vi "Test.vi"() -> ()   [LabVIEW 2020]
doc: "This VI is called when test mode begins, and will automatically be terminated when it ends. You can add manual or automatic tests and invoke them from the dashboard."
uses:
  <vilib>/Rock Robotics/WPI/ThirdParty/REV Robotics/REVLib/Typedef/Spark MAX Control Type.ctl
  <vilib>/Rock Robotics/WPI/Utilities/WPI_GetSetVariantRefNum.vi
  981LabViewComponents/2022 Robot Global Data.vi
panel:
  out "test telop\noutput\ncommand":dbl
  out "Error\n(armSetpoint -\n armPosition)":dbl
  out "Commanded\nSet Output":dbl
  out "Premove\nSensor Position":dbl
  out "Sensor Position 2":dbl
  out "armSetpoint":dbl
  out "Sensor Position":dbl
  out "x*y":dbl
  out "element":dbl
  out "x-y":dbl
  out "coerced(x) 2":dbl
  out "Position Error 2":dbl
  out "Position Error":dbl
  in  "PID Zero Constants":T1
  out "Status Plot":dbl[](graph)
  out "YRPHfH":T2
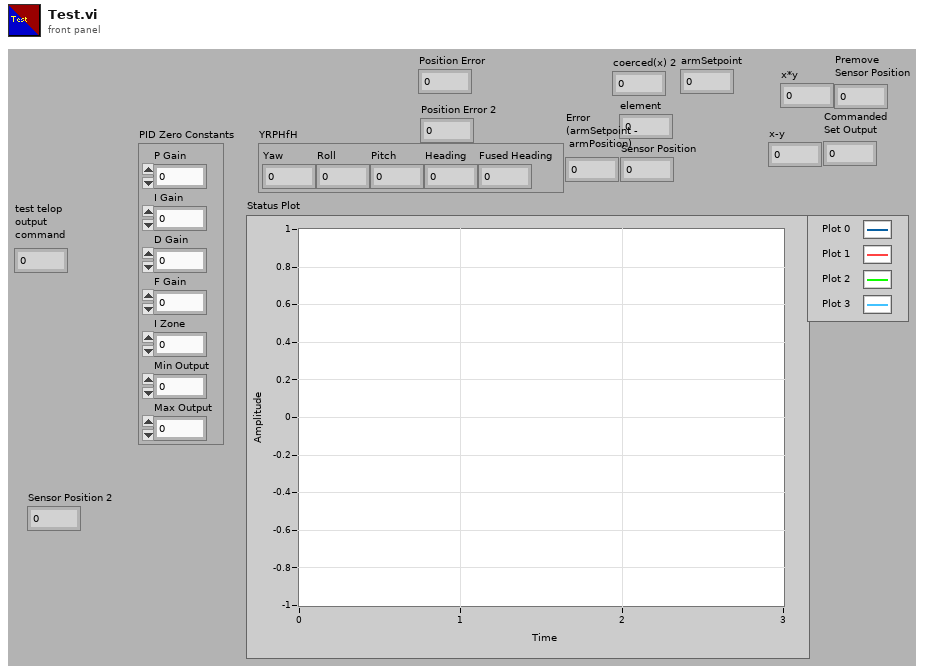
[diagram p1: front panel]
types:
  T1 = cluster{"P Gain":dbl, "I Gain":dbl, "D Gain":dbl, "F Gain":dbl, "I Zone":dbl, "Min Output":dbl, "Max Output":dbl}
  T2 = cluster{"Yaw":dbl, "Roll":dbl, "Pitch":dbl, "Heading":dbl, "Fused Heading":dbl}
  T3 = typedef "WPI_JoystickDevRef.ctl" = cluster{"Device":T4}
  T4 = typedef "WPI_JoystickDeviceEnum.ctl" = enum16{"USB 0", "USB 1", "USB 2", "USB 3", "USB 4", "USB 5"}
  T5 = typedef "WPI_MotorControlDeviceRef.ctl" = cluster{"DeviceStatus":errorcluster, "Type":T6, "PWM":cluster{"PWM Channel":T7, "DeadBand":T8}, "CAN":cluster{"Device Number":u8, "SetOutput VI Ref":variant, "GetOutput VI Ref":variant, "Enable VI Ref":variant, "Disable VI Ref":variant, "Data":variant}, "Invert":bool, "DIO PWM":cluster{"PWM \"Enable\" Channel":T7, "DIOChannel":T9, "PWM Rate":dbl}}
  T6 = typedef "WPI_MotorControlType.ctl" = enum16{"PWM", "CAN", "DIO PWM"}
  T7 = typedef "FPGA_DIOPWMChannel.ctl" = enum8{"PWM 0", "PWM 1", "PWM 2", "PWM 3", "PWM 4", "PWM 5", "PWM 6", "PWM 7", "PWM 8", "PWM 9", "PWM MXP 0", "PWM MXP 1", "PWM MXP 2", "PWM MXP 3", "PWM MXP 4", "PWM MXP 5", "PWM MXP 6", "PWM MXP 7", "PWM MXP 8", "PWM MXP 9", "Invalid"}
  T8 = typedef "WPI_PWMDeadband.ctl" = cluster{"Name":string, "maxPositivePwm":i32, "minPositivePwm":i32, "centerPwm":i32, "maxNegativePwm":i32, "minNegativePwm":i32, "angularRange":u16}
  T9 = typedef "FPGA_DIOChannel.ctl" = enum8{"DIO 0", "DIO 1", "DIO 2", "DIO 3", "DIO 4", "DIO 5", "DIO 6", "DIO 7", "DIO 8", "DIO 9", "DIO MXP 0", "DIO MXP 1", "DIO MXP 2", "DIO MXP 3", "DIO MXP 4", "DIO MXP 5", "DIO MXP 6", "DIO MXP 7", "DIO MXP 8", "DIO MXP 9", "DIO MXP 10", "DIO MXP 11", "DIO MXP 12", "DIO MXP 13", "DIO MXP 14", "DIO MXP 15", "SPI Port CS1", "SPI Port CS2", "SPI Port CS3", "SPI Port MISO", "SPI Port MOSI", "Invalid"}
  T10 = typedef "Spark MAX Control Type.ctl" = enum16{"Percent VBus", "Voltage", "Velocity", "Position", "Smart Motion", "Current", "Smart Velocity"}
  T11 = cluster{"P Gain":bool, "I Gain":bool, "D Gain":bool, "F Gain":bool, "I Zone":bool, "Min Output":bool, "Max Output":bool}
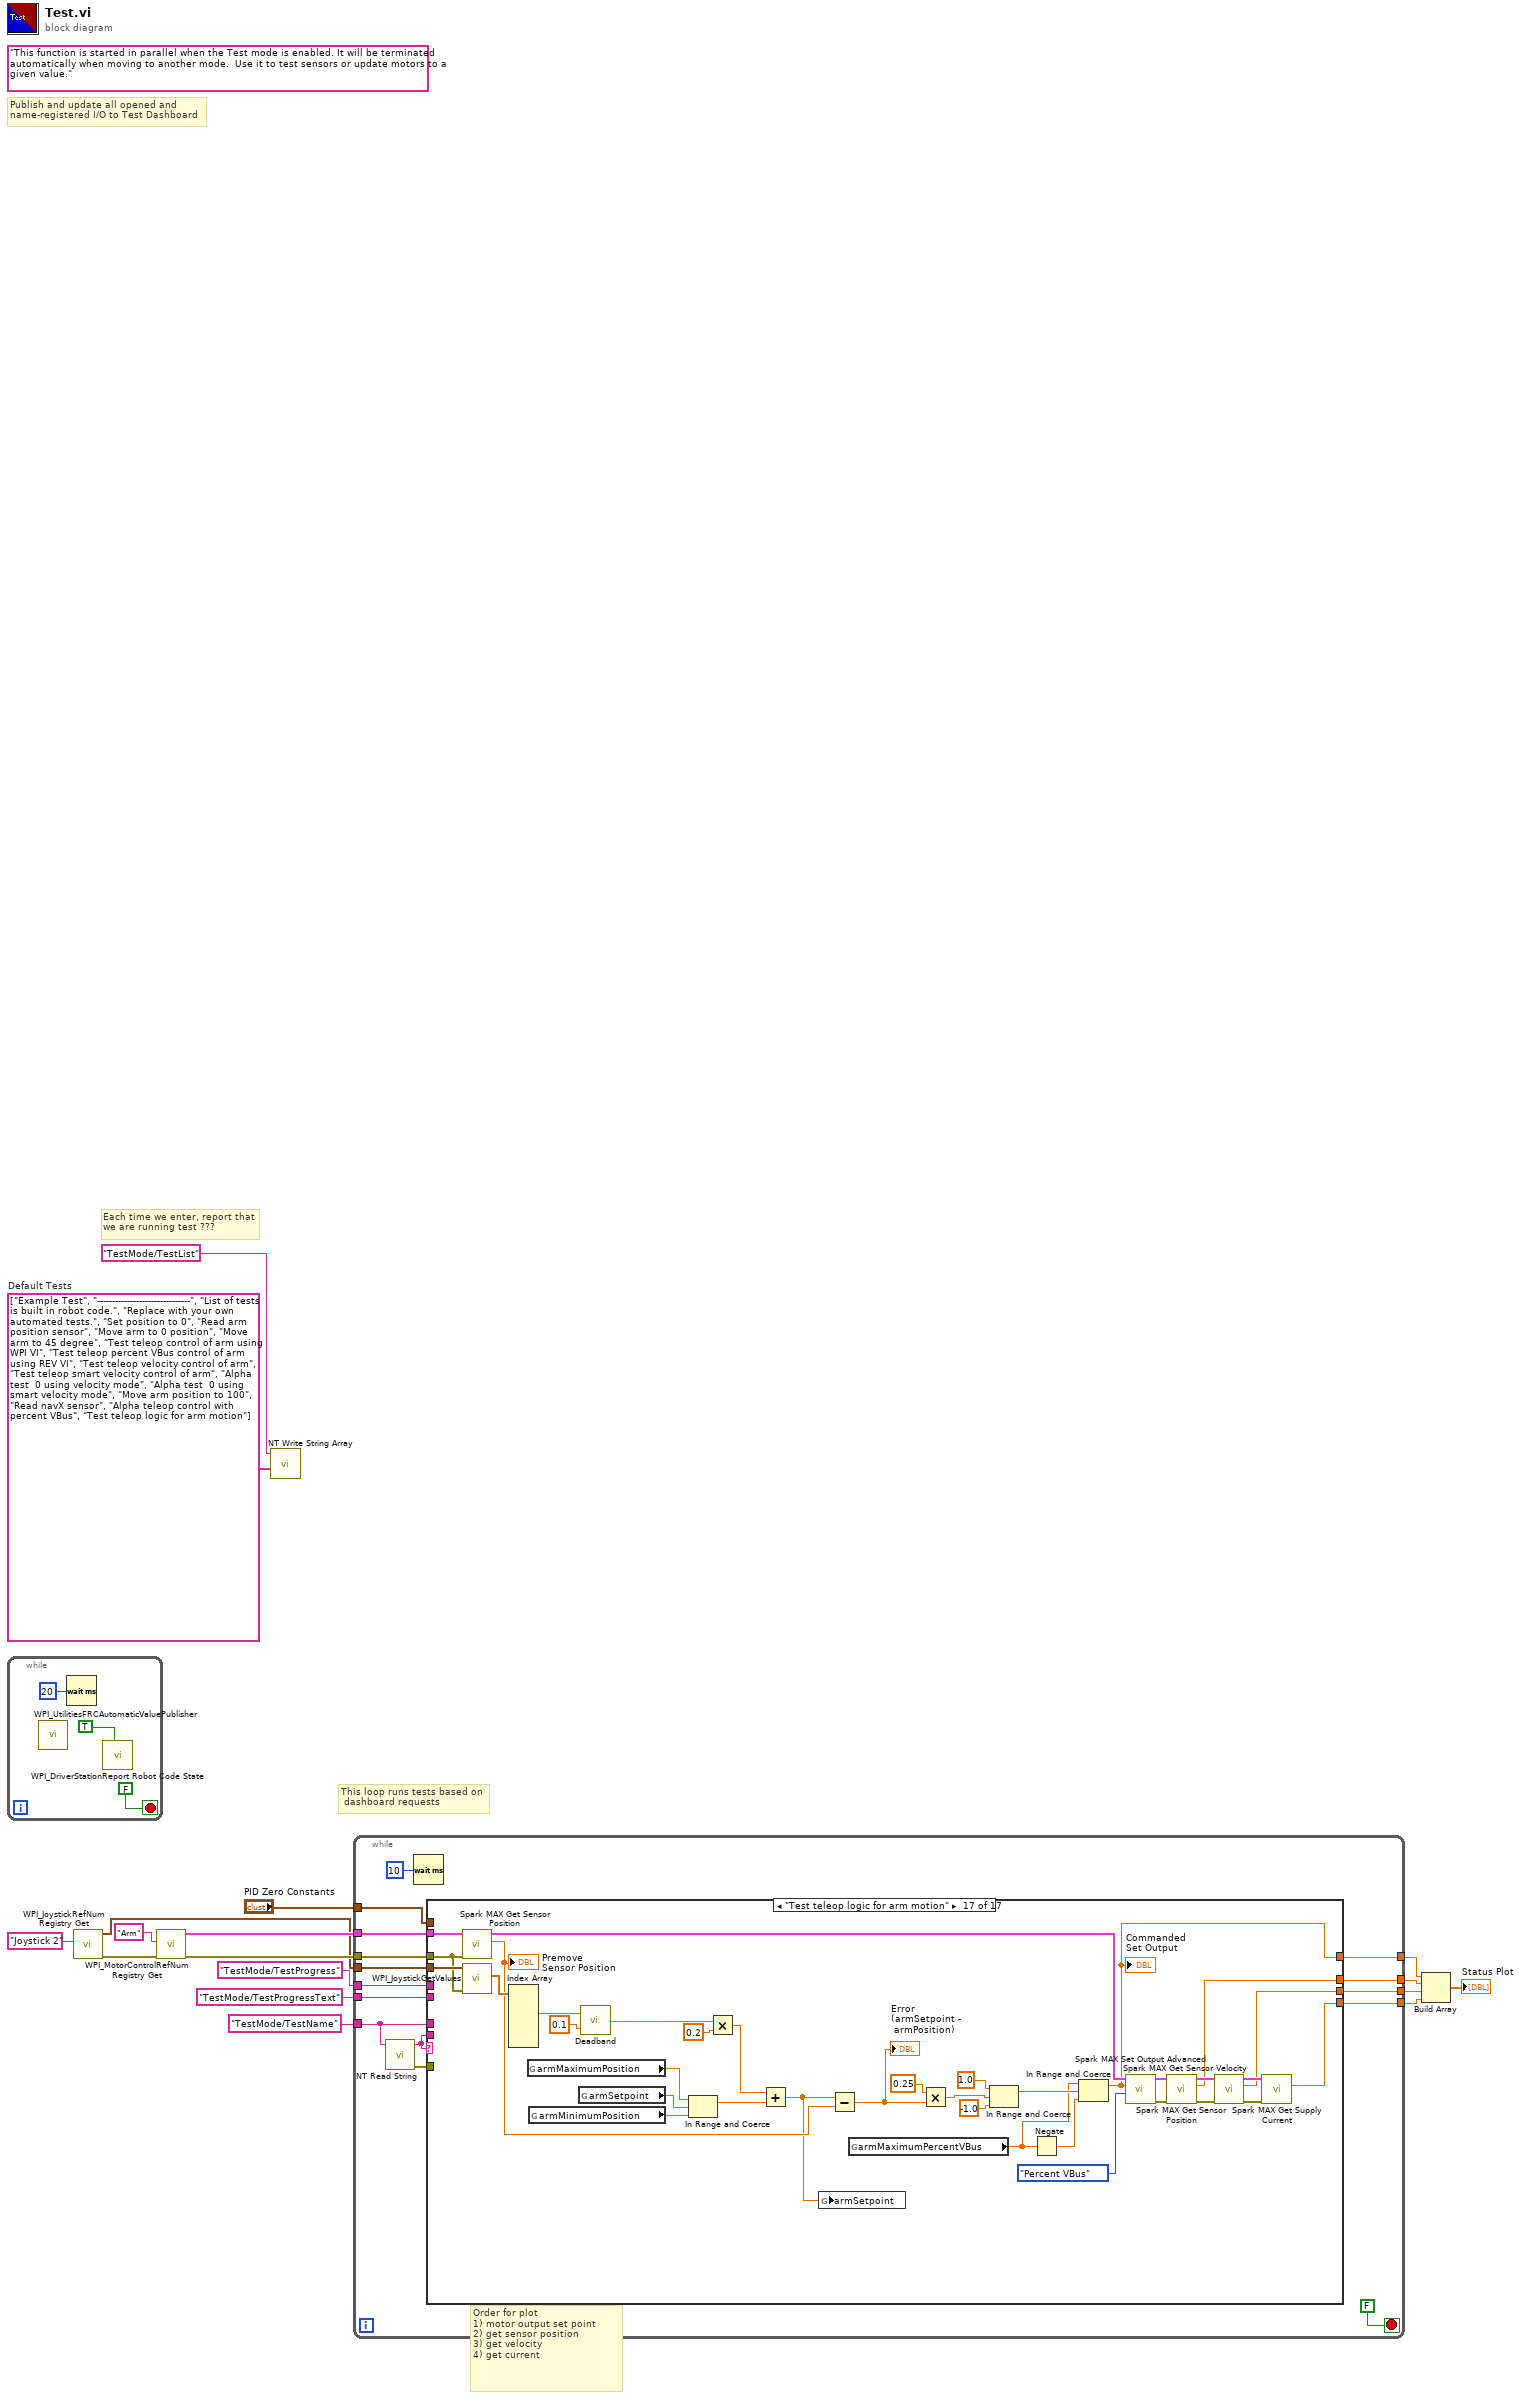
[diagram p0: block diagram]
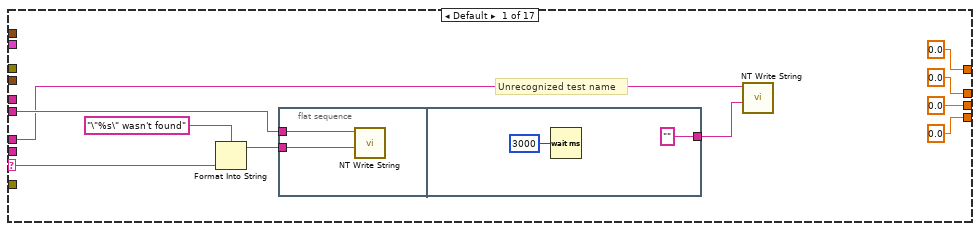
[diagram p2: hidden frame]
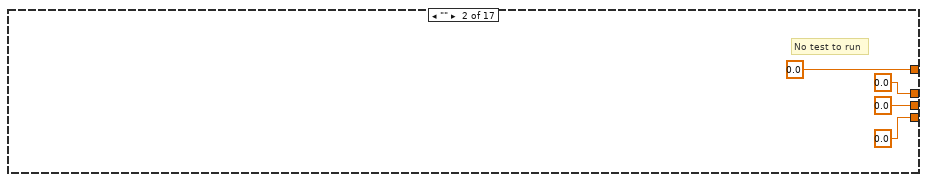
[diagram p3: hidden frame]
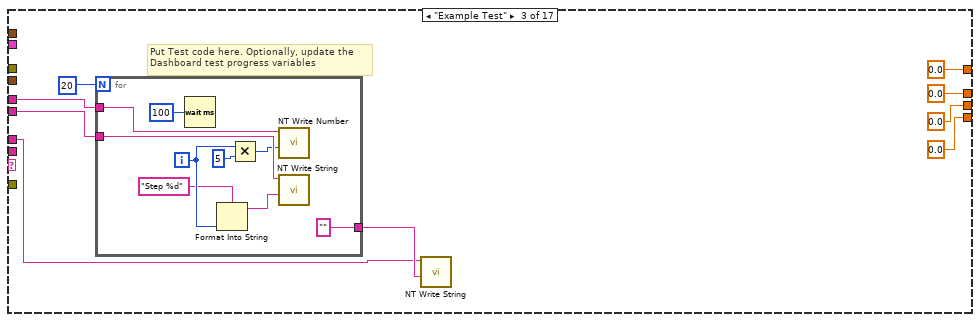
[diagram p4: hidden frame]
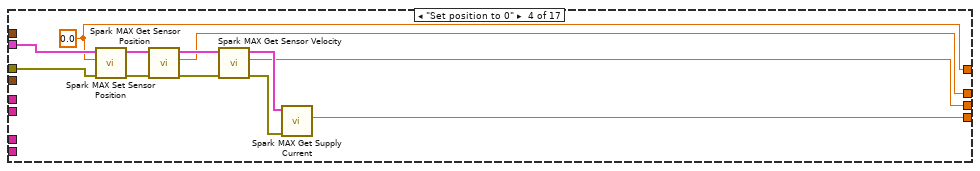
[diagram p5: hidden frame]
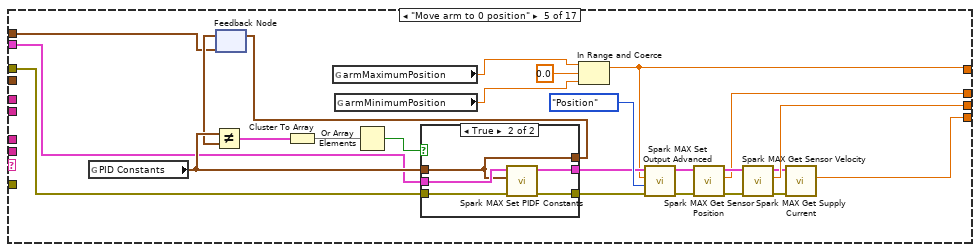
[diagram p6: hidden frame]
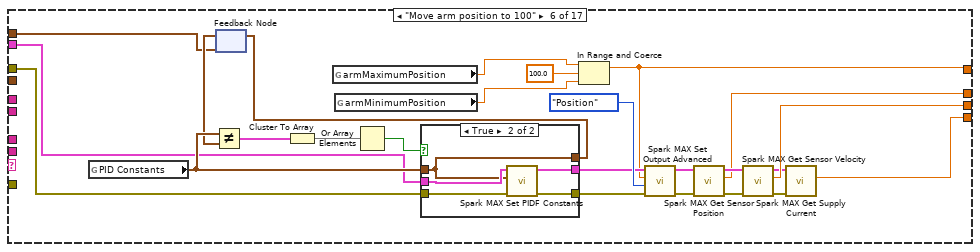
[diagram p8: hidden frame]
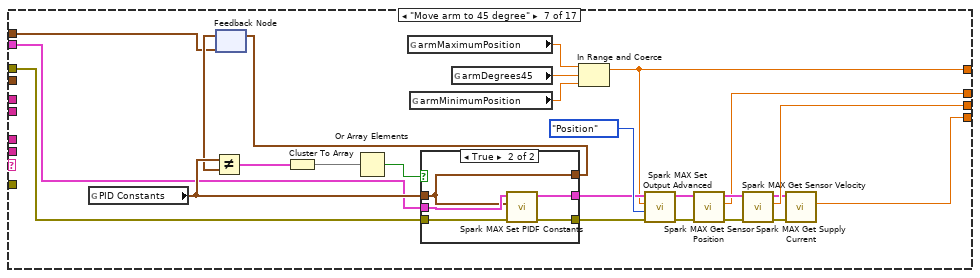
[diagram p10: hidden frame]
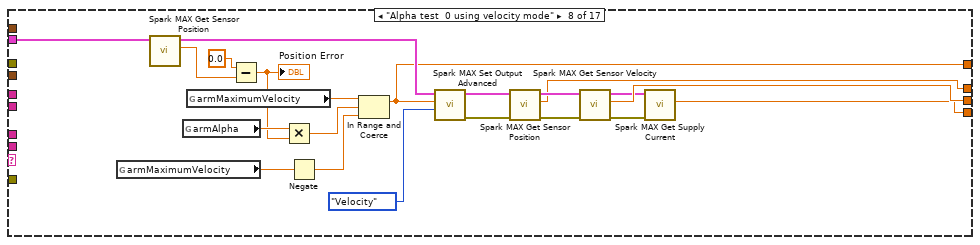
[diagram p12: hidden frame]
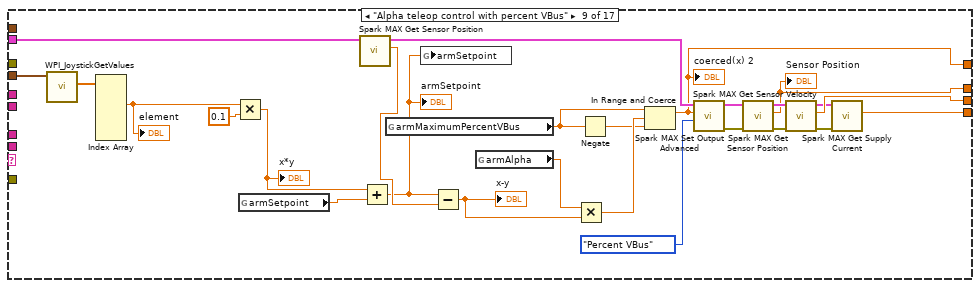
[diagram p13: hidden frame]
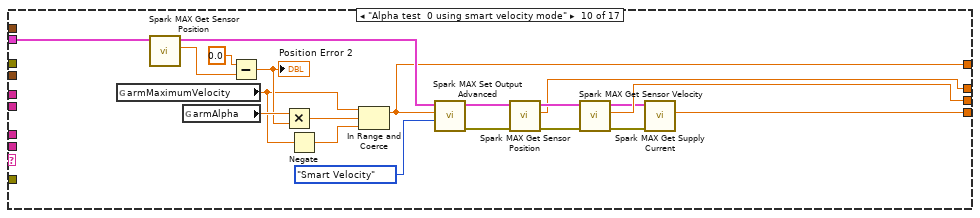
[diagram p14: hidden frame]
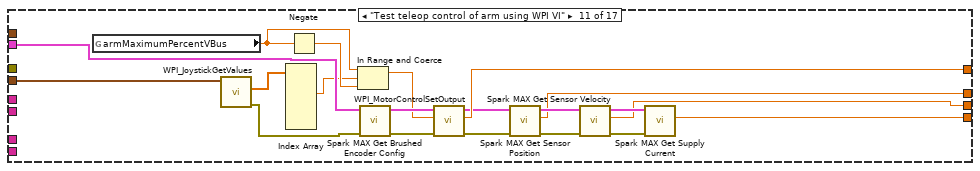
[diagram p15: hidden frame]
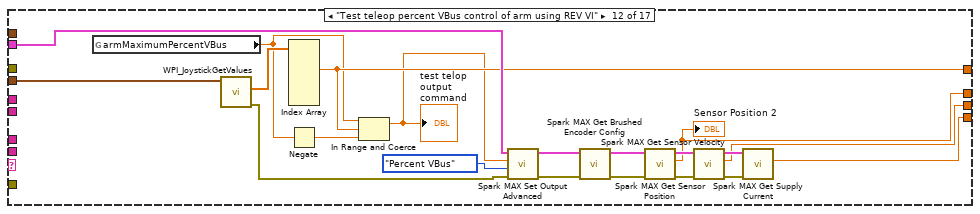
[diagram p16: hidden frame]
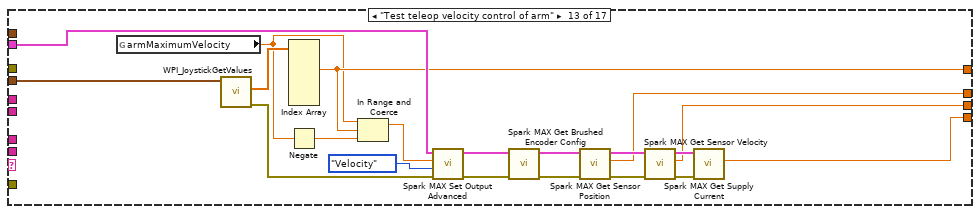
[diagram p17: hidden frame]
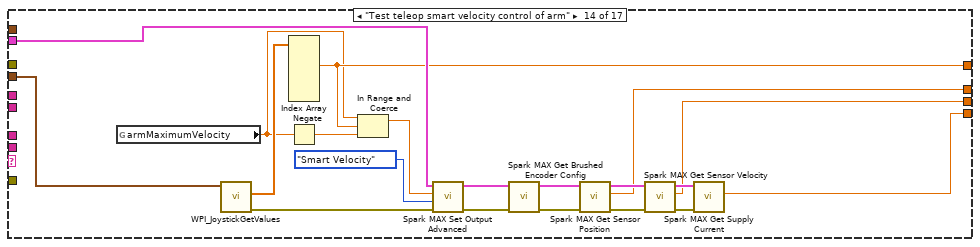
[diagram p18: hidden frame]
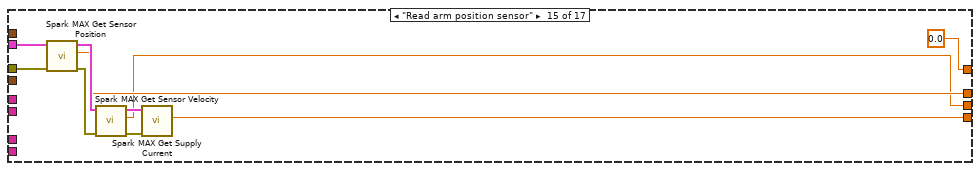
[diagram p19: hidden frame]
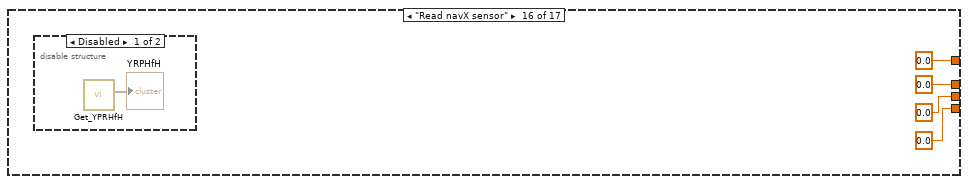
[diagram p20: hidden frame]
diagram:
  w14 = string[] ["Example Test", "-------------------------------", "List of tests is built in robot code.", "Replace with your own automated tests.", "Set position to 0", "Read arm position sensor", "Move arm to 0 position", "Move arm to 45 degree", "Test teleop control of arm using WPI VI", "Test teleop percent VBus control of arm using REV VI", "Test teleop velocity control of arm", "Test teleop smart velocity control of arm", "Alpha test  0 using velocity mode", "Alpha test  0 using smart velocity mode", "Move arm position to 100", "Read navX sensor", "Alpha teleop control with percent VBus", "Test teleop logic for arm motion"]  # Default Tests
  (unwired) "This function is started in parallel when the Test mode is enabled. It will be terminated automatically when moving to another mode.  Use it to test sensors or update motors to a given value."
  # "This loop runs tests based on \n dashboard requests"
  # "Publish and update all opened and\nname-registered I/O to Test Dashboard"
  # "Each time we enter, report that\nwe are running test ???"
  n1 = while {
    stop <- FALSE stop-if-true
    n2 = call <vilib>:"WPI_UtilitiesFRCAutomaticValuePublisher.vi"() -> ()  [unwired: 12 in]
    n3 = Wait (ms)(milliseconds to wait=u32 20) -> ()  [unwired: 1 out]
    n4 = call <vilib>:"WPI_DriverStationReport Robot Code State.vi"("Test"=TRUE ("Autonomous")) -> ()  [unwired: 10 in, 1 out]
  }
  n5 = call <vilib>:"WPI_JoystickRefNum Registry Get.vi"("refnum name"="Joystick 2") -> ("error out"=w1:errorcluster, "JoystickDevRef"=w7:T3)  [unwired: 1 in, 8 out]
  n6 = call <vilib>:"WPI_MotorControlRefNum Registry Get.vi"("error in (no error)"=w1, "refnum name"="Arm") -> ("error out"=w9:errorcluster, "MotorControlDevRef"=w10:T5)  [unwired: 8 in]
  n7 = call <vilib>:"NT Write String Array.vi"("String Array"=w14, "Name"="TestMode/TestList") -> ()  [unwired: 9 in, 1 out]
  n8 = while {
    tunnel: "TestMode/TestName" ("Name") -> [w30]
    tunnel: "TestMode/TestProgressText" ("Name") -> [w33]
    tunnel: "TestMode/TestProgress" ("Name") -> [w32]
    tunnel: w7 -> [w28]
    tunnel: w10 -> [w27]
    tunnel: w9 -> [w26]
    tunnel: "PID Zero Constants" -> [w25]
    tunnel: [w24] -> w5
    tunnel: [w23] -> w2
    tunnel: [w22] -> w4
    tunnel: [w21] -> w3
    stop <- FALSE stop-if-true
    # "Order for plot\n1) motor output set point\n2) get sensor position\n3) get velocity\n4) get current"
    n9 = call <vilib>:"NT Read String.vi"("Name"=w30) -> ("error out"=w29:errorcluster, "String"=w31:string)  [unwired: 9 in]
    n10 = Wait (ms)(milliseconds to wait=u32 10) -> ()  [unwired: 1 out]
    n11 = case shown="\"Test teleop logic for arm motion\"" w31 {
      selector: w31 -> [w44 _ _ _ _ _ _ _ _ _ _ _ _ _ _ _ _]
      tunnel: w30 -> [w41 _ w58 _ _ _ _ _ _ _ _ _ _ _ _ _ _]
      tunnel: w33 -> [w45 _ w61 _ _ _ _ _ _ _ _ _ _ _ _ _ _]
      tunnel: w32 -> [_ _ w62 _ _ _ _ _ _ _ _ _ _ _ _ _ _]
      tunnel: w31 -> [_ _ _ _ _ _ _ _ _ _ _ _ _ _ _ _ _]
      tunnel: w29 -> [_ _ _ _ _ _ _ _ _ _ _ _ _ _ _ _ _]
      tunnel: [0.0 ("armMaximumPosition") 0.0 ("armMaximumPosition") 0.0 ("armMaximumPosition") w81 w93 w126 w159 w183 w213 w231 w268 w273 w291 w312 0.0 ("armMaximumPosition") 0.0 ("armMaximumPosition") w349] -> w24
      tunnel: [0.0 ("Sensor Position") 0.0 ("Sensor Position") 0.0 ("Sensor Position") w73 w92 w125 w158 w200 w226 w246 w256 w270 w295 w315 w332 0.0 ("Sensor Position") w348] -> w23
      tunnel: [0.0 ("Sensor Velocity") 0.0 ("Sensor Velocity") 0.0 ("Sensor Velocity") w72 w91 w124 w157 w199 w225 w245 w255 w275 w294 w314 w331 0.0 ("Sensor Velocity") w347] -> w22
      tunnel: [0.0 ("Sensor Position") 0.0 ("Sensor Position") 0.0 ("Sensor Position") w80 w87 w120 w153 w196 w222 w242 w254 w282 w302 w322 w330 0.0 ("Sensor Position") w346] -> w21
      tunnel: w28 -> [_ _ _ _ _ _ _ _ w207 _ w267 w285 w305 w325 _ _ w374]
      tunnel: w27 -> [_ _ _ w83 w86 w119 w152 w191 w217 w237 w266 w284 w304 w324 w338 _ w373]
      tunnel: w26 -> [_ _ _ w82 w85 w118 w151 _ _ _ _ _ _ _ w339 _ w372]
      tunnel: w25 -> [_ _ _ _ w84 w117 w150 _ _ _ _ _ _ _ _ _ _]
      frame Default {
        # "Unrecognized test name"
        n12 = Format Into String(format string="\"%s\" wasn't found" ("Name"), w44) -> (resulting string=w43:string)  [unwired: 2 in, 1 out]
        n13 = flat-sequence {
          tunnel: w45 -> [w46]
          tunnel: w43 -> [w47]
          tunnel: ["" ("Name")] -> w40
          frame #0 {
            n14 = call <vilib>:"NT Write String.vi"("String"=w47, "Name"=w46) -> ()  [unwired: 9 in, 1 out]
          }
          frame #1 {
            n15 = Wait (ms)(milliseconds to wait=u32 3000) -> ()  [unwired: 1 out]
          }
        }
        n16 = call <vilib>:"NT Write String.vi"("String"=w40, "Name"=w41) -> ()  [unwired: 9 in, 1 out]
      }
      frame "" {
        # "No test to run"
      }
      frame "Example Test" {
        # "Put Test code here. Optionally, update the\nDashboard test progress variables"
        n17 = for {
          N: 20 -> [_]
          tunnel: w62 -> [w71]
          tunnel: w61 -> [w69]
          tunnel: ["" ("String")] -> w59
          i -> [w66]
          n18 = Wait (ms)(milliseconds to wait=u32 100) -> ()  [unwired: 1 out]
          n19 = Format Into String(format string="Step %d", w66) -> (resulting string=w64:string)  [unwired: 2 in, 1 out]
          n20 = Multiply(x=w66, y=u32 5 ("milliseconds to wait")) -> (x*y=w67:u32)
          n21 = call <vilib>:"NT Write Number.vi"("Numeric"=w67, "Name"=w71) -> ()  [unwired: 9 in, 1 out]
          n22 = call <vilib>:"NT Write String.vi"("String"=w64, "Name"=w69) -> ()  [unwired: 9 in, 1 out]
        }
        n23 = call <vilib>:"NT Write String.vi"("String"=w59, "Name"=w58) -> ()  [unwired: 9 in, 1 out]
      }
      frame "Set position to 0" {
        w81 = 0.0 ("Position")
        n24 = call <vilib>:"Spark MAX Set Sensor Position.vi"("error in"=w82, "Position"=w81, "MotorControlDeviceRef"=w83) -> ("error out"=w79:errorcluster, "MotorControlDeviceRef"=w78:T5)  [unwired: 7 in]
        n25 = call <vilib>:"Spark MAX Get Sensor Position.vi"("error in (no error)"=w79, "MotorControlDevRef in"=w78) -> ("error out"=w77:errorcluster, "Sensor Position"=w73:dbl, "MotorControlDevRef out"=w76:T5)  [unwired: 6 in, 1 out]
        n26 = call <vilib>:"Spark MAX Get Sensor Velocity.vi"("error in (no error)"=w77, "MotorControlDevRef in"=w76) -> ("error out"=w74:errorcluster, "Sensor Velocity"=w72:dbl, "MotorControlDevRef out"=w75:T5)  [unwired: 6 in, 1 out]
        n27 = call <vilib>:"Spark MAX Get Supply Current.vi"("error in (no error)"=w74, "MotorControlDevRef in"=w75) -> ("Current"=w80:dbl)  [unwired: 6 in, 3 out]
      }
      frame "Move arm to 0 position" {
        n28 = global read "2022 Robot Global Data.vi" "PID Constants"() -> (w99:T1)
        n29 = feedback #1(w84) -> (w98:T1)
        n30 = Not Equal?(x=w99, y=w98) -> (x != y?=w97:T11)
        n31 = Cluster To Array(cluster=w97) -> (array=w96:bool[])
        n32 = global read "2022 Robot Global Data.vi" "armMaximumPosition"() -> (w107:dbl)
        n33 = global read "2022 Robot Global Data.vi" "armMinimumPosition"() -> (w106:dbl)
        n34 = Or Array Elements(Boolean array=w96) -> (logical OR=w95:bool)
        n35 = case shown="True" w95 {
          tunnel: w85 -> [w109 w116]
          tunnel: w86 -> [w110 w115]
          tunnel: [w109 w114] -> w101
          tunnel: [w110 w113] -> w100
          tunnel: w99 -> [w111 w112]
          tunnel: [w111 w112] -> w94
          frame False {
          }
          frame True {
            n36 = call <vilib>:"Spark MAX Set PIDF Constants.vi"("error in"=w116, "PID Constants"=w112, "MotorControlDeviceRef"=w115) -> ("error out"=w114:errorcluster, "MotorControlDeviceRef"=w113:T5)  [unwired: 7 in]
          }
        }
        n37 = feedback-in #1(w94) -> ()
        n38 = In Range and Coerce(upper limit=w107, x=0.0, lower limit=w106) -> (coerced(x)=w93:dbl)  [unwired: 1 out]
        n39 = call <vilib>:"Spark MAX Set Output Advanced.vi"("error in (no error)"=w101, "Control Mode"=Spark_MAX_Control_Type."Position", "Setpoint"=w93, "MotorControlDevRef"=w100) -> ("error out"=w105:errorcluster, "MotorControlDevRef"=w103:T5)  [unwired: 6 in]
        n40 = call <vilib>:"Spark MAX Get Sensor Position.vi"("error in (no error)"=w105, "MotorControlDevRef in"=w103) -> ("error out"=w104:errorcluster, "Sensor Position"=w92:dbl, "MotorControlDevRef out"=w102:T5)  [unwired: 6 in, 1 out]
        n41 = call <vilib>:"Spark MAX Get Sensor Velocity.vi"("error in (no error)"=w104, "MotorControlDevRef in"=w102) -> ("error out"=w88:errorcluster, "Sensor Velocity"=w91:dbl, "MotorControlDevRef out"=w89:T5)  [unwired: 6 in, 1 out]
        n42 = call <vilib>:"Spark MAX Get Supply Current.vi"("error in (no error)"=w88, "MotorControlDevRef in"=w89) -> ("Current"=w87:dbl)  [unwired: 6 in, 3 out]
      }
      frame "Move arm position to 100" {
        n43 = global read "2022 Robot Global Data.vi" "PID Constants"() -> (w132:T1)
        n44 = feedback #2(w117) -> (w131:T1)
        n45 = Not Equal?(x=w132, y=w131) -> (x != y?=w130:T11)
        n46 = Cluster To Array(cluster=w130) -> (array=w129:bool[])
        n47 = global read "2022 Robot Global Data.vi" "armMaximumPosition"() -> (w140:dbl)
        n48 = global read "2022 Robot Global Data.vi" "armMinimumPosition"() -> (w139:dbl)
        n49 = Or Array Elements(Boolean array=w129) -> (logical OR=w128:bool)
        n50 = case shown="True" w128 {
          tunnel: w118 -> [w142 w149]
          tunnel: w119 -> [w143 w148]
          tunnel: [w142 w147] -> w134
          tunnel: [w143 w146] -> w133
          tunnel: w132 -> [w144 w145]
          tunnel: [w144 w145] -> w127
          frame False {
          }
          frame True {
            n51 = call <vilib>:"Spark MAX Set PIDF Constants.vi"("error in"=w149, "PID Constants"=w145, "MotorControlDeviceRef"=w148) -> ("error out"=w147:errorcluster, "MotorControlDeviceRef"=w146:T5)  [unwired: 7 in]
          }
        }
        n52 = feedback-in #2(w127) -> ()
        n53 = In Range and Coerce(upper limit=w140, x=100.0, lower limit=w139) -> (coerced(x)=w126:dbl)  [unwired: 1 out]
        n54 = call <vilib>:"Spark MAX Set Output Advanced.vi"("error in (no error)"=w134, "Control Mode"=Spark_MAX_Control_Type."Position", "Setpoint"=w126, "MotorControlDevRef"=w133) -> ("error out"=w138:errorcluster, "MotorControlDevRef"=w136:T5)  [unwired: 6 in]
        n55 = call <vilib>:"Spark MAX Get Sensor Position.vi"("error in (no error)"=w138, "MotorControlDevRef in"=w136) -> ("error out"=w137:errorcluster, "Sensor Position"=w125:dbl, "MotorControlDevRef out"=w135:T5)  [unwired: 6 in, 1 out]
        n56 = call <vilib>:"Spark MAX Get Sensor Velocity.vi"("error in (no error)"=w137, "MotorControlDevRef in"=w135) -> ("error out"=w121:errorcluster, "Sensor Velocity"=w124:dbl, "MotorControlDevRef out"=w122:T5)  [unwired: 6 in, 1 out]
        n57 = call <vilib>:"Spark MAX Get Supply Current.vi"("error in (no error)"=w121, "MotorControlDevRef in"=w122) -> ("Current"=w120:dbl)  [unwired: 6 in, 3 out]
      }
      frame "Move arm to 45 degree" {
        n58 = global read "2022 Robot Global Data.vi" "PID Constants"() -> (w164:T1)
        n59 = feedback #3(w150) -> (w163:T1)
        n60 = Not Equal?(x=w164, y=w163) -> (x != y?=w162:T11)
        n61 = Cluster To Array(cluster=w162) -> (array=w161:bool[])
        n62 = Or Array Elements(Boolean array=w161) -> (logical OR=w160:bool)
        n63 = global read "2022 Robot Global Data.vi" "armMaximumPosition"() -> (w173:dbl)
        n64 = global read "2022 Robot Global Data.vi" "armMinimumPosition"() -> (w172:dbl)
        n65 = case shown="True" w160 {
          tunnel: w151 -> [w175 w182]
          tunnel: w152 -> [w176 w181]
          tunnel: [w175 w180] -> w166
          tunnel: [w176 w179] -> w165
          tunnel: w164 -> [w177 w178]
          tunnel: [w177 w178] -> w156
          frame False {
          }
          frame True {
            n66 = call <vilib>:"Spark MAX Set PIDF Constants.vi"("error in"=w182, "PID Constants"=w178, "MotorControlDeviceRef"=w181) -> ("error out"=w180:errorcluster, "MotorControlDeviceRef"=w179:T5)  [unwired: 7 in]
          }
        }
        n67 = feedback-in #3(w156) -> ()
        n68 = global read "2022 Robot Global Data.vi" "armDegrees45"() -> (w171:dbl)
        n69 = In Range and Coerce(upper limit=w173, x=w171, lower limit=w172) -> (coerced(x)=w159:dbl)  [unwired: 1 out]
        n70 = call <vilib>:"Spark MAX Set Output Advanced.vi"("error in (no error)"=w166, "Control Mode"=Spark_MAX_Control_Type."Position", "Setpoint"=w159, "MotorControlDevRef"=w165) -> ("error out"=w170:errorcluster, "MotorControlDevRef"=w168:T5)  [unwired: 6 in]
        n71 = call <vilib>:"Spark MAX Get Sensor Position.vi"("error in (no error)"=w170, "MotorControlDevRef in"=w168) -> ("error out"=w169:errorcluster, "Sensor Position"=w158:dbl, "MotorControlDevRef out"=w167:T5)  [unwired: 6 in, 1 out]
        n72 = call <vilib>:"Spark MAX Get Sensor Velocity.vi"("error in (no error)"=w169, "MotorControlDevRef in"=w167) -> ("error out"=w154:errorcluster, "Sensor Velocity"=w157:dbl, "MotorControlDevRef out"=w155:T5)  [unwired: 6 in, 1 out]
        n73 = call <vilib>:"Spark MAX Get Supply Current.vi"("error in (no error)"=w154, "MotorControlDevRef in"=w155) -> ("Current"=w153:dbl)  [unwired: 6 in, 3 out]
      }
      frame "Alpha test  0 using velocity mode" {
        n74 = global read "2022 Robot Global Data.vi" "armMaximumVelocity"() -> (w186:dbl)
        n75 = call <vilib>:"Spark MAX Get Sensor Position.vi"("MotorControlDevRef in"=w191) -> ("Sensor Position"=w194:dbl, "MotorControlDevRef out"=w190:T5)  [unwired: 7 in, 2 out]
        n76 = global read "2022 Robot Global Data.vi" "armAlpha"() -> (w193:dbl)
        n77 = global read "2022 Robot Global Data.vi" "armMaximumVelocity"() -> (w187:dbl)
        n78 = Subtract(x=0.0, y=w194) -> (x-y=w192:dbl)
        "Position Error" <- w192
        n79 = Multiply(x=w193, y=w192) -> (x*y=w184:dbl)
        n80 = Negate(x=w186) -> (-x=w185:dbl)
        n81 = In Range and Coerce(upper limit=w187, x=w184, lower limit=w185) -> (coerced(x)=w183:dbl)  [unwired: 1 out]
        n82 = call <vilib>:"Spark MAX Set Output Advanced.vi"("Control Mode"=Spark_MAX_Control_Type."Velocity", "Setpoint"=w183, "MotorControlDevRef"=w190) -> ("error out"=w188:errorcluster, "MotorControlDevRef"=w189:T5)  [unwired: 7 in]
        n83 = call <vilib>:"Spark MAX Get Sensor Position.vi"("error in (no error)"=w188, "MotorControlDevRef in"=w189) -> ("error out"=w202:errorcluster, "Sensor Position"=w200:dbl, "MotorControlDevRef out"=w201:T5)  [unwired: 6 in, 1 out]
        n84 = call <vilib>:"Spark MAX Get Sensor Velocity.vi"("error in (no error)"=w202, "MotorControlDevRef in"=w201) -> ("error out"=w197:errorcluster, "Sensor Velocity"=w199:dbl, "MotorControlDevRef out"=w198:T5)  [unwired: 6 in, 1 out]
        n85 = call <vilib>:"Spark MAX Get Supply Current.vi"("error in (no error)"=w197, "MotorControlDevRef in"=w198) -> ("Current"=w196:dbl)  [unwired: 6 in, 3 out]
      }
      frame "Alpha teleop control with percent VBus" {
        n86 = call <vilib>:"WPI_JoystickGetValues.vi"("JoystickDevRef"=w207) -> ("Axes"=w212:dbl[])  [unwired: 6 in, 4 out]
        n87 = Index Array(array=w212) -> (element #2=w206:dbl)  [unwired: 6 in, 5 out]
        "element" <- w206
        n88 = Multiply(x=w206, y=0.1) -> (x*y=w210:dbl)
        "x*y" <- w210
        n89 = global read "2022 Robot Global Data.vi" "armSetpoint"() -> (w209:dbl)
        n90 = call <vilib>:"Spark MAX Get Sensor Position.vi"("MotorControlDevRef in"=w217) -> ("Sensor Position"=w221:dbl, "MotorControlDevRef out"=w216:T5)  [unwired: 7 in, 2 out]
        n91 = Add(x=w210, y=w209) -> (x+y=w208:dbl)
        "armSetpoint" <- w208
        n92 = global read "2022 Robot Global Data.vi" "armMaximumPercentVBus"() -> (w204:dbl)
        n93 = global write "2022 Robot Global Data.vi" "armSetpoint"(w208) -> ()
        n94 = Subtract(x=w208, y=w221) -> (x-y=w219:dbl)
        "x-y" <- w219
        n95 = global read "2022 Robot Global Data.vi" "armAlpha"() -> (w220:dbl)
        n96 = Multiply(x=w220, y=w219) -> (x*y=w218:dbl)
        n97 = Negate(x=w204) -> (-x=w205:dbl)
        n98 = In Range and Coerce(upper limit=w204, x=w218, lower limit=w205) -> (coerced(x)=w213:dbl)  [unwired: 1 out]
        "coerced(x) 2" <- w213
        n99 = call <vilib>:"Spark MAX Set Output Advanced.vi"("Control Mode"=Spark_MAX_Control_Type."Percent VBus", "Setpoint"=w213, "MotorControlDevRef"=w216) -> ("error out"=w214:errorcluster, "MotorControlDevRef"=w215:T5)  [unwired: 7 in]
        n100 = call <vilib>:"Spark MAX Get Sensor Position.vi"("error in (no error)"=w214, "MotorControlDevRef in"=w215) -> ("error out"=w228:errorcluster, "Sensor Position"=w226:dbl, "MotorControlDevRef out"=w227:T5)  [unwired: 6 in, 1 out]
        "Sensor Position" <- w226
        n101 = call <vilib>:"Spark MAX Get Sensor Velocity.vi"("error in (no error)"=w228, "MotorControlDevRef in"=w227) -> ("error out"=w223:errorcluster, "Sensor Velocity"=w225:dbl, "MotorControlDevRef out"=w224:T5)  [unwired: 6 in, 1 out]
        n102 = call <vilib>:"Spark MAX Get Supply Current.vi"("error in (no error)"=w223, "MotorControlDevRef in"=w224) -> ("Current"=w222:dbl)  [unwired: 6 in, 3 out]
      }
      frame "Alpha test  0 using smart velocity mode" {
        n103 = global read "2022 Robot Global Data.vi" "armMaximumVelocity"() -> (w230:dbl)
        n104 = call <vilib>:"Spark MAX Get Sensor Position.vi"("MotorControlDevRef in"=w237) -> ("Sensor Position"=w240:dbl, "MotorControlDevRef out"=w236:T5)  [unwired: 7 in, 2 out]
        n105 = global read "2022 Robot Global Data.vi" "armAlpha"() -> (w239:dbl)
        n106 = Subtract(x=0.0, y=w240) -> (x-y=w238:dbl)
        "Position Error 2" <- w238
        n107 = Multiply(x=w239, y=w238) -> (x*y=w232:dbl)
        n108 = Negate(x=w230) -> (-x=w233:dbl)
        n109 = In Range and Coerce(upper limit=w230, x=w232, lower limit=w233) -> (coerced(x)=w231:dbl)  [unwired: 1 out]
        n110 = call <vilib>:"Spark MAX Set Output Advanced.vi"("Control Mode"=Spark_MAX_Control_Type."Smart Velocity", "Setpoint"=w231, "MotorControlDevRef"=w236) -> ("error out"=w234:errorcluster, "MotorControlDevRef"=w235:T5)  [unwired: 7 in]
        n111 = call <vilib>:"Spark MAX Get Sensor Position.vi"("error in (no error)"=w234, "MotorControlDevRef in"=w235) -> ("error out"=w248:errorcluster, "Sensor Position"=w246:dbl, "MotorControlDevRef out"=w247:T5)  [unwired: 6 in, 1 out]
        n112 = call <vilib>:"Spark MAX Get Sensor Velocity.vi"("error in (no error)"=w248, "MotorControlDevRef in"=w247) -> ("error out"=w243:errorcluster, "Sensor Velocity"=w245:dbl, "MotorControlDevRef out"=w244:T5)  [unwired: 6 in, 1 out]
        n113 = call <vilib>:"Spark MAX Get Supply Current.vi"("error in (no error)"=w243, "MotorControlDevRef in"=w244) -> ("Current"=w242:dbl)  [unwired: 6 in, 3 out]
      }
      frame "Test teleop control of arm using WPI VI" {
        n114 = global read "2022 Robot Global Data.vi" "armMaximumPercentVBus"() -> (w250:dbl)
        n115 = call <vilib>:"WPI_JoystickGetValues.vi"("JoystickDevRef"=w267) -> ("error out"=w265:errorcluster, "Axes"=w269:dbl[])  [unwired: 6 in, 3 out]
        n116 = Index Array(array=w269) -> (element #2=w252:dbl)  [unwired: 6 in, 5 out]
        n117 = Negate(x=w250) -> (-x=w253:dbl)
        n118 = In Range and Coerce(upper limit=w250, x=w252, lower limit=w253) -> (coerced(x)=w251:dbl)  [unwired: 1 out]
        n119 = call <vilib>:"Spark MAX Get Brushed Encoder Config.vi"("error in (no error)"=w265, "MotorControlDeviceRef in"=w266) -> ("error out"=w263:errorcluster, "MotorControlDeviceRef"=w264:T5)  [unwired: 4 in, 4 out]
        n120 = call <vilib>:"WPI_MotorControlSetOutput.vi"("error in (no error)"=w263, "Output"=w251, "MotorControlDevRef"=w264) -> ("error out"=w262:errorcluster, "Motor Output"=w268:dbl, "MotorControlDevRef"=w259:T5)  [unwired: 6 in]
        n121 = call <vilib>:"Spark MAX Get Sensor Position.vi"("error in (no error)"=w262, "MotorControlDevRef in"=w259) -> ("error out"=w261:errorcluster, "Sensor Position"=w256:dbl, "MotorControlDevRef out"=w258:T5)  [unwired: 6 in, 1 out]
        n122 = call <vilib>:"Spark MAX Get Sensor Velocity.vi"("error in (no error)"=w261, "MotorControlDevRef in"=w258) -> ("error out"=w260:errorcluster, "Sensor Velocity"=w255:dbl, "MotorControlDevRef out"=w257:T5)  [unwired: 6 in, 1 out]
        n123 = call <vilib>:"Spark MAX Get Supply Current.vi"("error in (no error)"=w260, "MotorControlDevRef in"=w257) -> ("Current"=w254:dbl)  [unwired: 6 in, 3 out]
      }
      frame "Test teleop percent VBus control of arm using REV VI" {
        n124 = global read "2022 Robot Global Data.vi" "armMaximumPercentVBus"() -> (w271:dbl)
        n125 = call <vilib>:"WPI_JoystickGetValues.vi"("JoystickDevRef"=w285) -> ("error out"=w283:errorcluster, "Axes"=w289:dbl[])  [unwired: 6 in, 3 out]
        n126 = Index Array(array=w289) -> (element #2=w273:dbl)  [unwired: 6 in, 5 out]
        n127 = Negate(x=w271) -> (-x=w274:dbl)
        n128 = In Range and Coerce(upper limit=w271, x=w273, lower limit=w274) -> (coerced(x)=w272:dbl)  [unwired: 1 out]
        "test telop\noutput\ncommand" <- w272
        n129 = call <vilib>:"Spark MAX Set Output Advanced.vi"("error in (no error)"=w283, "Control Mode"=Spark_MAX_Control_Type."Percent VBus", "Setpoint"=w272, "MotorControlDevRef"=w284) -> ("error out"=w286:errorcluster, "MotorControlDevRef"=w287:T5)  [unwired: 6 in]
        n130 = call <vilib>:"Spark MAX Get Brushed Encoder Config.vi"("error in (no error)"=w286, "MotorControlDeviceRef in"=w287) -> ("error out"=w278:errorcluster, "MotorControlDeviceRef"=w281:T5)  [unwired: 4 in, 4 out]
        n131 = call <vilib>:"Spark MAX Get Sensor Position.vi"("error in (no error)"=w278, "MotorControlDevRef in"=w281) -> ("error out"=w277:errorcluster, "Sensor Position"=w270:dbl, "MotorControlDevRef out"=w280:T5)  [unwired: 6 in, 1 out]
        "Sensor Position 2" <- w270
        n132 = call <vilib>:"Spark MAX Get Sensor Velocity.vi"("error in (no error)"=w277, "MotorControlDevRef in"=w280) -> ("error out"=w276:errorcluster, "Sensor Velocity"=w275:dbl, "MotorControlDevRef out"=w279:T5)  [unwired: 6 in, 1 out]
        n133 = call <vilib>:"Spark MAX Get Supply Current.vi"("error in (no error)"=w276, "MotorControlDevRef in"=w279) -> ("Current"=w282:dbl)  [unwired: 6 in, 3 out]
      }
      frame "Test teleop velocity control of arm" {
        n134 = global read "2022 Robot Global Data.vi" "armMaximumVelocity"() -> (w290:dbl)
        n135 = call <vilib>:"WPI_JoystickGetValues.vi"("JoystickDevRef"=w305) -> ("error out"=w303:errorcluster, "Axes"=w309:dbl[])  [unwired: 6 in, 3 out]
        n136 = Index Array(array=w309) -> (element #2=w291:dbl)  [unwired: 6 in, 5 out]
        n137 = Negate(x=w290) -> (-x=w293:dbl)
        n138 = In Range and Coerce(upper limit=w290, x=w291, lower limit=w293) -> (coerced(x)=w292:dbl)  [unwired: 1 out]
        n139 = call <vilib>:"Spark MAX Set Output Advanced.vi"("error in (no error)"=w303, "Control Mode"=Spark_MAX_Control_Type."Velocity", "Setpoint"=w292, "MotorControlDevRef"=w304) -> ("error out"=w306:errorcluster, "MotorControlDevRef"=w307:T5)  [unwired: 6 in]
        n140 = call <vilib>:"Spark MAX Get Brushed Encoder Config.vi"("error in (no error)"=w306, "MotorControlDeviceRef in"=w307) -> ("error out"=w298:errorcluster, "MotorControlDeviceRef"=w301:T5)  [unwired: 4 in, 4 out]
        n141 = call <vilib>:"Spark MAX Get Sensor Position.vi"("error in (no error)"=w298, "MotorControlDevRef in"=w301) -> ("error out"=w297:errorcluster, "Sensor Position"=w295:dbl, "MotorControlDevRef out"=w300:T5)  [unwired: 6 in, 1 out]
        n142 = call <vilib>:"Spark MAX Get Sensor Velocity.vi"("error in (no error)"=w297, "MotorControlDevRef in"=w300) -> ("error out"=w296:errorcluster, "Sensor Velocity"=w294:dbl, "MotorControlDevRef out"=w299:T5)  [unwired: 6 in, 1 out]
        n143 = call <vilib>:"Spark MAX Get Supply Current.vi"("error in (no error)"=w296, "MotorControlDevRef in"=w299) -> ("Current"=w302:dbl)  [unwired: 6 in, 3 out]
      }
      frame "Test teleop smart velocity control of arm" {
        n144 = global read "2022 Robot Global Data.vi" "armMaximumVelocity"() -> (w310:dbl)
        n145 = call <vilib>:"WPI_JoystickGetValues.vi"("JoystickDevRef"=w325) -> ("error out"=w323:errorcluster, "Axes"=w329:dbl[])  [unwired: 6 in, 3 out]
        n146 = Index Array(array=w329) -> (element #2=w312:dbl)  [unwired: 6 in, 5 out]
        n147 = Negate(x=w310) -> (-x=w313:dbl)
        n148 = In Range and Coerce(upper limit=w310, x=w312, lower limit=w313) -> (coerced(x)=w311:dbl)  [unwired: 1 out]
        n149 = call <vilib>:"Spark MAX Set Output Advanced.vi"("error in (no error)"=w323, "Control Mode"=Spark_MAX_Control_Type."Smart Velocity", "Setpoint"=w311, "MotorControlDevRef"=w324) -> ("error out"=w326:errorcluster, "MotorControlDevRef"=w327:T5)  [unwired: 6 in]
        n150 = call <vilib>:"Spark MAX Get Brushed Encoder Config.vi"("error in (no error)"=w326, "MotorControlDeviceRef in"=w327) -> ("error out"=w318:errorcluster, "MotorControlDeviceRef"=w321:T5)  [unwired: 4 in, 4 out]
        n151 = call <vilib>:"Spark MAX Get Sensor Position.vi"("error in (no error)"=w318, "MotorControlDevRef in"=w321) -> ("error out"=w317:errorcluster, "Sensor Position"=w315:dbl, "MotorControlDevRef out"=w320:T5)  [unwired: 6 in, 1 out]
        n152 = call <vilib>:"Spark MAX Get Sensor Velocity.vi"("error in (no error)"=w317, "MotorControlDevRef in"=w320) -> ("error out"=w316:errorcluster, "Sensor Velocity"=w314:dbl, "MotorControlDevRef out"=w319:T5)  [unwired: 6 in, 1 out]
        n153 = call <vilib>:"Spark MAX Get Supply Current.vi"("error in (no error)"=w316, "MotorControlDevRef in"=w319) -> ("Current"=w322:dbl)  [unwired: 6 in, 3 out]
      }
      frame "Read arm position sensor" {
        n154 = call <vilib>:"Spark MAX Get Sensor Position.vi"("error in (no error)"=w339, "MotorControlDevRef in"=w338) -> ("error out"=w336:errorcluster, "Sensor Position"=w332:dbl, "MotorControlDevRef out"=w337:T5)  [unwired: 6 in, 1 out]
        n155 = call <vilib>:"Spark MAX Get Sensor Velocity.vi"("error in (no error)"=w336, "MotorControlDevRef in"=w337) -> ("error out"=w334:errorcluster, "Sensor Velocity"=w331:dbl, "MotorControlDevRef out"=w335:T5)  [unwired: 6 in, 1 out]
        n156 = call <vilib>:"Spark MAX Get Supply Current.vi"("error in (no error)"=w334, "MotorControlDevRef in"=w335) -> ("Current"=w330:dbl)  [unwired: 6 in, 3 out]
      }
      frame "Read navX sensor" {
        n157 = disable-structure shown="Disabled" {
          frame Disabled {
            n158 = call <vilib>:"Get_YPRHfH.vi"() -> ("YRPHfH"=→"YRPHfH":T2)  [unwired: 11 in]
          }
          frame Enabled {
          }
        }
      }
      frame "Test teleop logic for arm motion" {
        n159 = call <vilib>:"Spark MAX Get Sensor Position.vi"("error in (no error)"=w372, "MotorControlDevRef in"=w373) -> ("Sensor Position"=w361:dbl, "MotorControlDevRef out"=w353:T5)  [unwired: 6 in, 2 out]
        "Premove\nSensor Position" <- w361
        n160 = call <vilib>:"WPI_JoystickGetValues.vi"("error in (no error)"=w372, "JoystickDevRef"=w374) -> ("Axes"=w379:dbl[])  [unwired: 5 in, 4 out]
        n161 = Index Array(array=w379) -> (element #2=w376:dbl)  [unwired: 6 in, 5 out]
        n162 = global read "2022 Robot Global Data.vi" "armMaximumPosition"() -> (w370:dbl)
        n163 = global read "2022 Robot Global Data.vi" "armMinimumPosition"() -> (w371:dbl)
        n164 = global read "2022 Robot Global Data.vi" "armSetpoint"() -> (w369:dbl)
        n165 = call "Deadband.vi"("Limit"=0.1, "Input"=w376) -> ("Output"=w375:dbl)
        n166 = In Range and Coerce(upper limit=w370, x=w369, lower limit=w371) -> (coerced(x)=w367:dbl)  [unwired: 1 out]
        n167 = Multiply(x=w375, y=0.2) -> (x*y=w368:dbl)
        n168 = Add(x=w368, y=w367) -> (x+y=w360:dbl)
        n169 = global write "2022 Robot Global Data.vi" "armSetpoint"(w360) -> ()
        n170 = Subtract(x=w360, y=w361) -> (x-y=w366:dbl)
        "Error\n(armSetpoint -\n armPosition)" <- w366
        n171 = global read "2022 Robot Global Data.vi" "armMaximumPercentVBus"() -> (w345:dbl)
        n172 = Multiply(x=0.25, y=w366) -> (x*y=w363:dbl)
        n173 = In Range and Coerce(upper limit=1.0, x=w363, lower limit=-1.0) -> (coerced(x)=w352:dbl)  [unwired: 1 out]
        n174 = Negate(x=w345) -> (-x=w351:dbl)
        n175 = In Range and Coerce(upper limit=w345, x=w352, lower limit=w351) -> (coerced(x)=w349:dbl)  [unwired: 1 out]
        "Commanded\nSet Output" <- w349
        n176 = call <vilib>:"Spark MAX Set Output Advanced.vi"("Control Mode"=Spark_MAX_Control_Type."Percent VBus", "Setpoint"=w349, "MotorControlDevRef"=w353) -> ("error out"=w354:errorcluster, "MotorControlDevRef"=w355:T5)  [unwired: 7 in]
        n177 = call <vilib>:"Spark MAX Get Sensor Position.vi"("error in (no error)"=w354, "MotorControlDevRef in"=w355) -> ("error out"=w359:errorcluster, "Sensor Position"=w348:dbl, "MotorControlDevRef out"=w358:T5)  [unwired: 6 in, 1 out]
        n178 = call <vilib>:"Spark MAX Get Sensor Velocity.vi"("error in (no error)"=w359, "MotorControlDevRef in"=w358) -> ("error out"=w356:errorcluster, "Sensor Velocity"=w347:dbl, "MotorControlDevRef out"=w357:T5)  [unwired: 6 in, 1 out]
        n179 = call <vilib>:"Spark MAX Get Supply Current.vi"("error in (no error)"=w356, "MotorControlDevRef in"=w357) -> ("Current"=w346:dbl)  [unwired: 6 in, 3 out]
      }
    }
  }
  n180 = Build Array(w5, w2, w4, w3) -> (→"Status Plot":dbl[])
